vi "move1.vi"(4 "error in (no error)":errorcluster, 6 "names":string[](array[string]), 7 "dir path":path) -> (0 "error out":errorcluster)   [LabVIEW 2010]
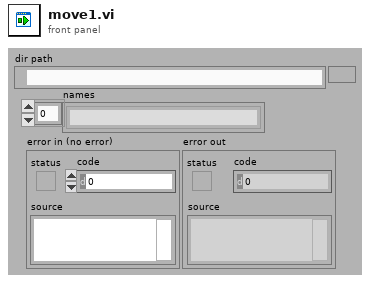
[diagram p1: front panel]
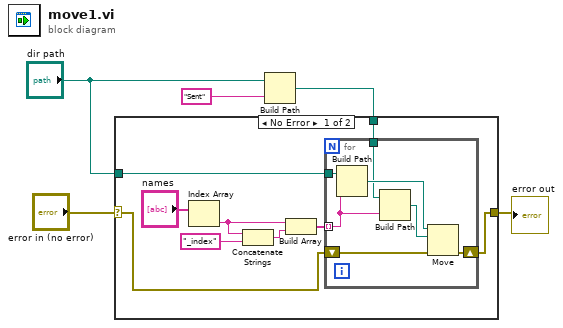
[diagram p0: block diagram]
diagram:
  n1 = Build Path(base path="dir path", name or relative path="Sent") -> (appended path=w1:path)
  n2 = case shown="No Error" "error in (no error)" {
    selector: "error in (no error)" -> [w9 w22]
    tunnel: [w8 w22] -> w5
    tunnel: "dir path" -> [w7 _]
    tunnel: w1 -> [w6 _]
    frame No Error {
      n3 = Index Array(array="names") -> (element=w11:string)  [unwired: 1 in]
      n4 = Concatenate Strings(w11, "_index" ("string")) -> (w12:string)
      n5 = Build Array(w11, w12) -> (w10:string[])
      n6 = for {
        tunnel: w10 -> [w15] mode=indexing
        tunnel: w7 -> [w21]
        shift-right: [w19] -> w8
        shift-left: w9 -> [w20]
        tunnel: w6 -> [w16]
        n7 = Build Path(base path=w21, name or relative path=w15) -> (appended path=w18:path)
        n8 = Build Path(base path=w16, name or relative path=w15) -> (appended path=w17:path)
        n9 = Move(source path=w18, error in=w20, 10:w17) -> (error out=w19:errorcluster)  [unwired: 2 in, 2 out]
      }
    }
    frame Error {
    }
  }
  "error out" <- w5
